vi "hangman.vi"() -> ()   [LabVIEW 2016]
panel:
  out "?":bool
  out "?":bool
  out "?":bool
  out "?":bool
  out "?":bool
  out "?":bool
  out "?":bool
  out "?":bool
  out "?":bool
  out "?":bool
  out "?":bool
  out "?":bool
  out "?":bool
  out "?":bool
  out "?":bool
  out "?":bool
  out "?":bool
  out "?":bool
  out "?":bool
  out "?":bool
  out "?":bool
  out "?":bool
  out "?":bool
  out "?":bool
  out "?":bool
  out "?":bool
  out "?":bool
  out "?":bool
  out "?":bool
  out "?":bool
  out "Wrong attempts":i32
  out "Too many letters":bool=TRUE
  out "Letters used":string
  out "?":string[](array[string])
  in  "?":bool
  in  "?":bool
  out "Word in \narray form":string[](array[string])
  out "Word Number":dbl
  out "Correct":bool
  out "Word":string
  in  "Enter Letter":string
  out "Path":path
  # "Created by: MartiniDesignz\nDate:            11/28/18"
  # "Under this is the correct word"
  # "Created by: MartiniDesignz\nDate:            11/28/18"
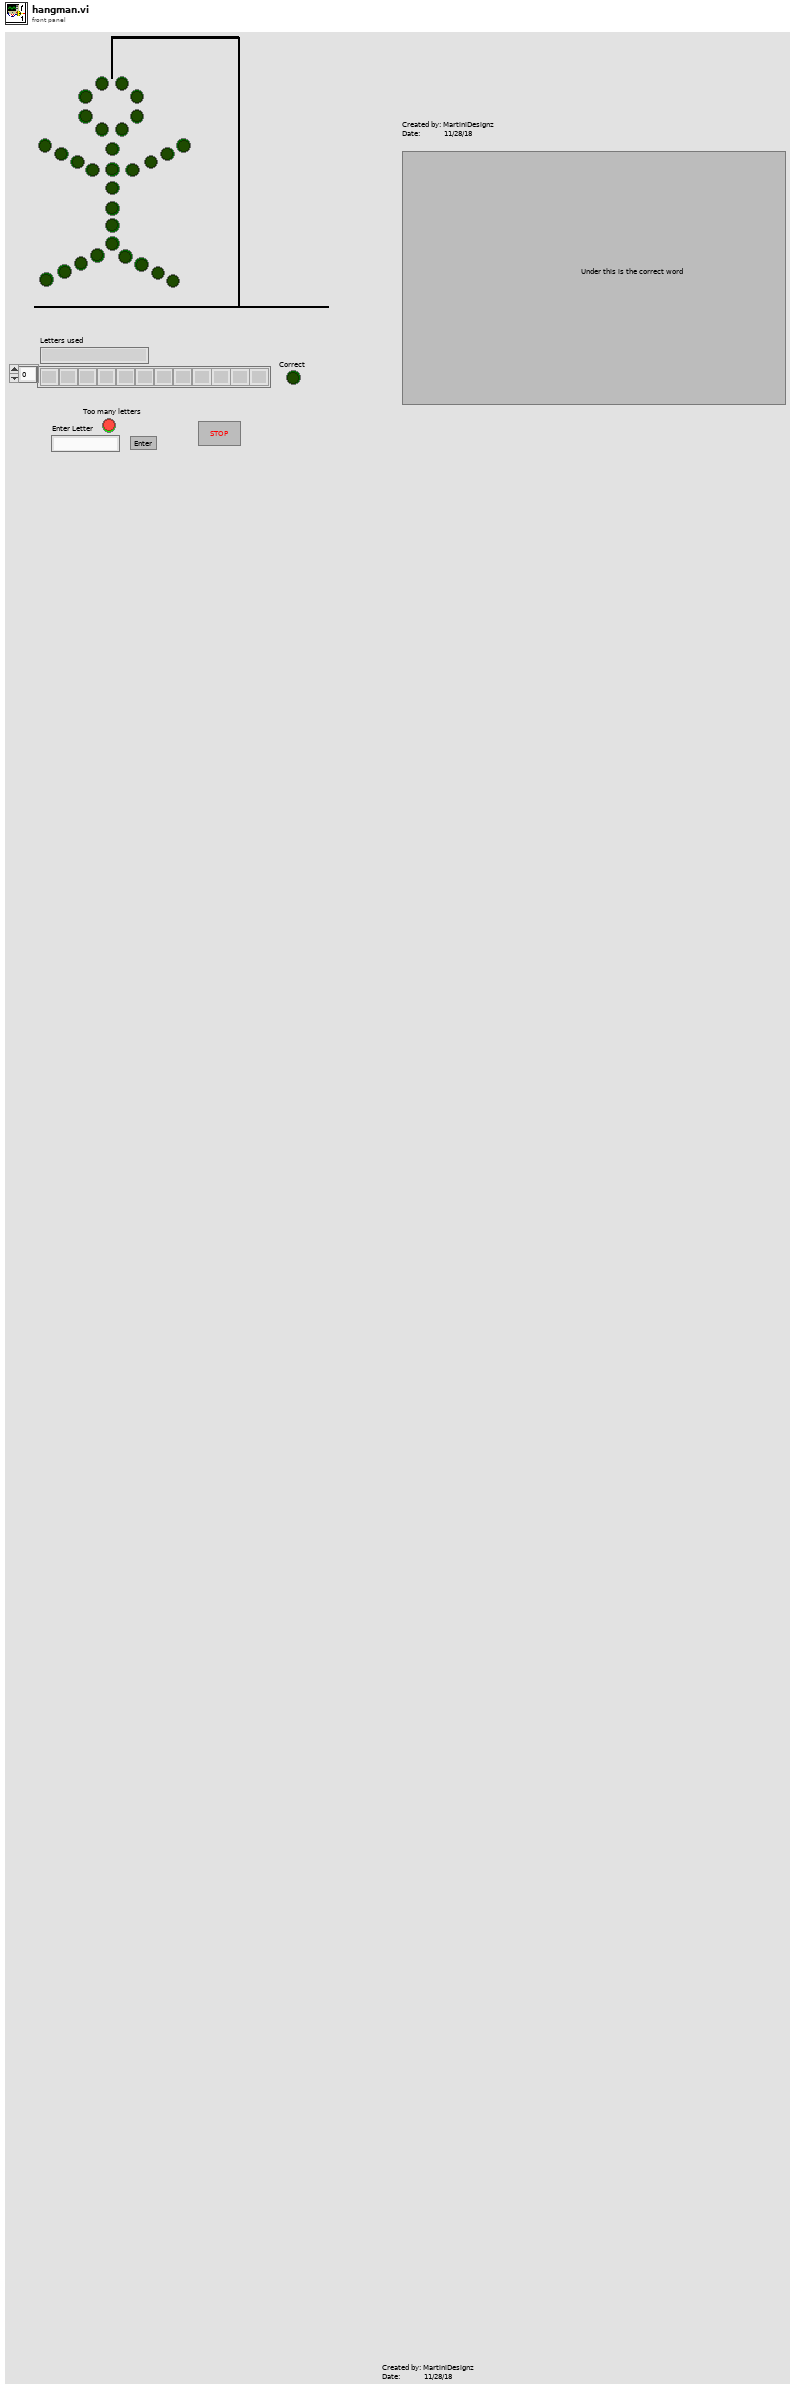
[diagram p1: front panel]
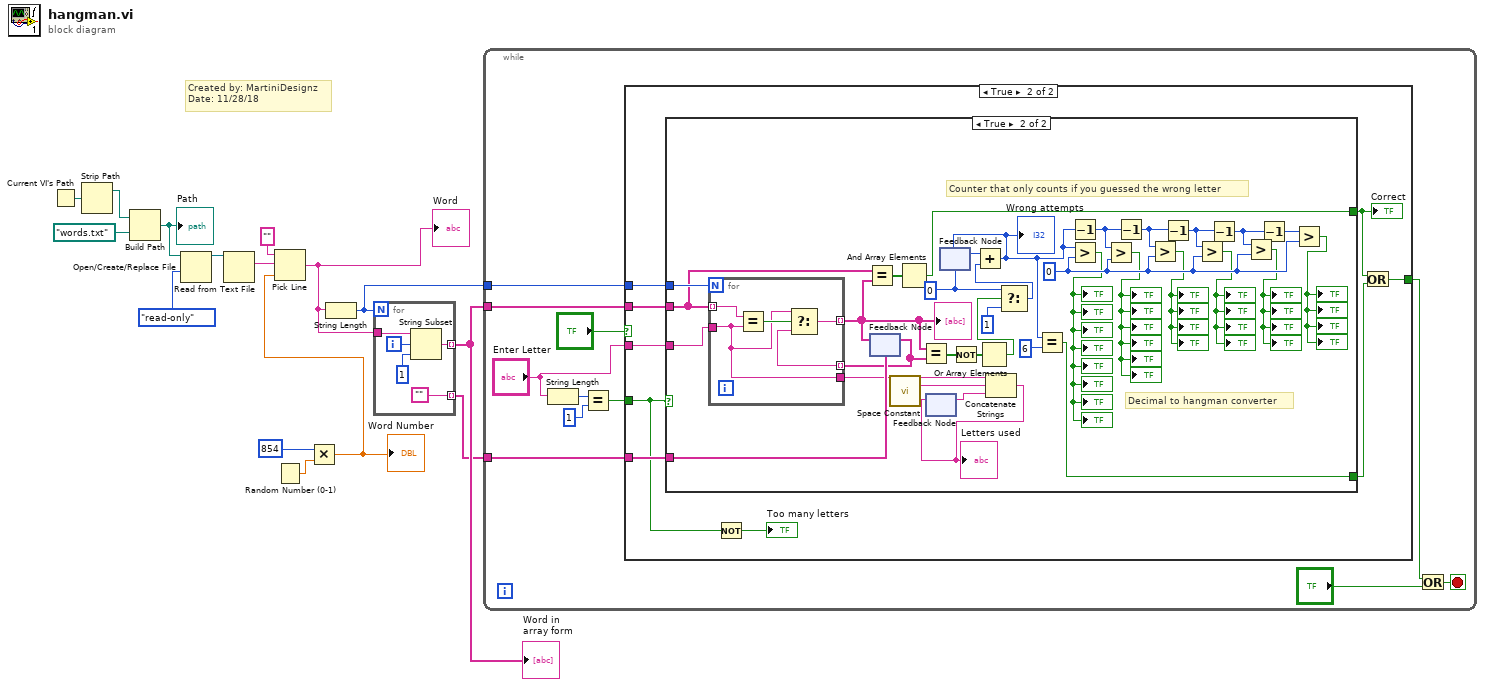
[diagram p0: block diagram]
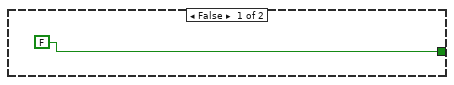
[diagram p2: hidden frame]
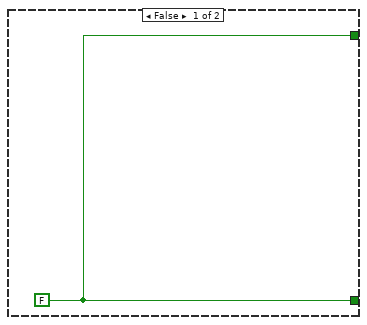
[diagram p3: hidden frame]
diagram:
  # "Created by: MartiniDesignz\nDate: 11/28/18"
  n1 = Current VI's Path() -> (path=w1:path)
  n2 = Strip Path(path=w1) -> (stripped path=w2:path)  [unwired: 1 out]
  n3 = Build Path(base path=w2, name or relative path=path "words.txt" ("file path (use dialog)")) -> (appended path=w4:path)
  "Path" <- w4
  n4 = Open/Create/Replace File(file path (use dialog)=w4, access (0:read/write)=enum16{"read/write", "read-only", "write-only"}."read-only") -> (refnum out=w8:refnum<file>)  [unwired: 4 in, 2 out]
  n5 = Read from Text File(file (use dialog)=w8) -> (text=w9:string)  [unwired: 3 in, 3 out]
  n6 = Random Number (0-1)() -> (number: 0 to 1=w14:dbl)
  n7 = Multiply(x=854, y=w14) -> (x*y=w6:dbl)
  "Word Number" <- w6
  n8 = Pick Line(string ("")="", multi-line string=w9, line index=w6) -> (output string=w10:string)
  "Word" <- w10
  n9 = String Length(string=w10) -> (length=w12:i32)
  n10 = for {
    N: w12 -> [_]
    tunnel: w10 -> [w20]
    tunnel: [w18] -> w11 mode=indexing
    tunnel: [""] -> w7 mode=indexing
    i -> [w16]
    n11 = String Subset(string=w20, offset (0)=w16, length (rest)=1) -> (substring=w18:string)
  }
  "Word in \narray form" <- w11
  n12 = while {
    tunnel: w12 -> [w25]
    tunnel: w11 -> [w26]
    tunnel: w7 -> [w24]
    stop <- w21 stop-if-true
    n13 = String Length(string="Enter Letter") -> (length=w28:i32)
    n14 = Equal?(x=w28, y=1) -> (x = y?=w27:bool)
    n15 = case shown="True" "?" {
      tunnel: w25 -> [_ w33]
      tunnel: w26 -> [_ w34]
      tunnel: "Enter Letter" -> [_ w35]
      tunnel: w24 -> [_ w37]
      tunnel: w27 -> [_ w36]
      tunnel: [FALSE w40] -> w22
      frame False {
      }
      frame True {
        n16 = case shown="True" w36 {
          tunnel: w33 -> [_ w76]
          tunnel: w34 -> [_ w53]
          tunnel: w35 -> [_ w52]
          tunnel: w37 -> [_ w75]
          tunnel: [w42 w70] -> w41
          tunnel: [w42 w61] -> w39
          frame False {
            w42 = FALSE
          }
          frame True {
            w56 = 0
            w64 = 0
            # "Decimal to hangman converter"
            # "Counter that only counts if you guessed the wrong letter"
            n17 = feedback #1(w75) -> (w69:string[])
            n18 = for {
              N: w76 -> [_]
              tunnel: w53 -> [w81] mode=indexing
              tunnel: w52 -> [w77]
              tunnel: [w80] -> w62 mode=indexing
              tunnel: w69 -> [w79] mode=indexing
              tunnel: [w77] -> w74
              n19 = Equal?(x=w81, y=w77) -> (x = y?=w78:bool)
              n20 = Select(t=w77, s=w78, f=w79) -> (s? t:f=w80:string)
            }
            "?" <- w62
            n21 = Equal?(x=w53, y=w62) -> (x = y?=w51:bool[])
            n22 = feedback-in #1(w62) -> ()
            n23 = call <vilib>:"Space Constant.vi"() -> ("String"=w72:string)
            n24 = And Array Elements(Boolean array=w51) -> (logical AND=w61:bool)
            n25 = Equal?(x=w62, y=w69) -> (x = y?=w65:bool[])
            n26 = feedback #2() -> (w73:string)  [unwired: 1 in]
            n27 = feedback #3(w64) -> (w67:i32)
            n28 = Not(x=w65) -> (.not. x?=w66:bool[])
            n29 = Or Array Elements(Boolean array=w66) -> (logical OR=w50:bool)
            n30 = Concatenate Strings(w74, w72, w73) -> (w49:string)
            "Letters used" <- w49
            n31 = feedback-in #2(w49) -> ()
            n32 = Select(t=w64, s=w50, f=1) -> (s? t:f=w68:i32)
            n33 = Add(x=w67, y=w68) -> (x+y=w60:i32)
            "Wrong attempts" <- w60
            n34 = feedback-in #3(w60) -> ()
            n35 = Equal?(x=w60, y=6) -> (x = y?=w70:bool)
            n36 = Decrement(x=w60) -> (x-1=w54:i32)
            n37 = Greater?(x=w60, y=w56) -> (0:→"?" →"?" →"?" →"?" →"?" →"?" →"?" →"?":bool)
            n38 = Greater?(x=w54, y=w56) -> (0:→"?" →"?" →"?" →"?" →"?" →"?":bool)
            n39 = Decrement(x=w54) -> (x-1=w59:i32)
            n40 = Greater?(x=w59, y=w56) -> (0:→"?" →"?" →"?" →"?":bool)
            n41 = Decrement(x=w59) -> (x-1=w58:i32)
            n42 = Greater?(x=w58, y=w56) -> (0:→"?" →"?" →"?" →"?":bool)
            n43 = Decrement(x=w58) -> (x-1=w55:i32)
            n44 = Greater?(x=w55, y=w56) -> (0:→"?" →"?" →"?" →"?":bool)
            n45 = Decrement(x=w55) -> (x-1=w57:i32)
            n46 = Greater?(x=w57, y=w56) -> (0:→"?" →"?" →"?" →"?":bool)
          }
        }
        "Correct" <- w39
        n47 = Not(x=w36) -> (.not. x?=→"Too many letters":bool)
        n48 = Or(x=w39, y=w41) -> (x .or. y?=w40:bool)
      }
    }
    n49 = Or(x=w22, y="?") -> (x .or. y?=w21:bool)
  }
